vi "Noise_Out_DI.vi"(5 "D2":bool, 6 "D1":bool, 7 "IN":dbl(slide) scale=0.0..9000.0) -> (0 "cluster":cluster{"[0]":dbl, "[1]":dbl}, 1 "DOUT_2":bool, 2 "DOUT_1":bool, 3 "OUT":u32)   [LabVIEW 2017]
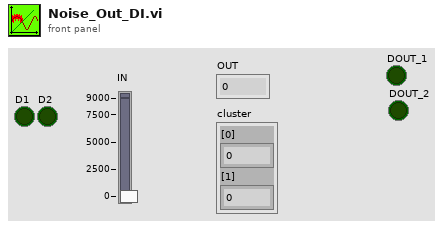
[diagram p1: front panel]
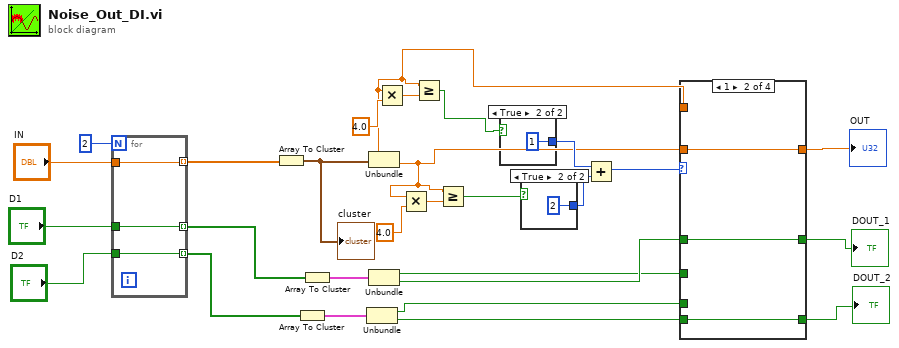
[diagram p0: block diagram]
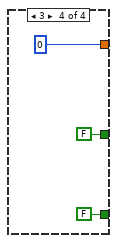
[diagram p4: hidden frame]
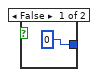
[diagram p5: hidden frame]
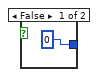
[diagram p6: hidden frame]
diagram:
  n1 = for {
    N: 2 -> [_]
    tunnel: [w31] -> w21 mode=indexing
    tunnel: "IN" -> [w31]
    tunnel: [w30] -> w18 mode=indexing
    tunnel: "D1" -> [w30]
    tunnel: [w29] -> w17 mode=indexing
    tunnel: "D2" -> [w29]
  }
  n2 = Array To Cluster(array=w21) -> (cluster=w28:cluster{"[0]":dbl, "[1]":dbl})
  "cluster" <- w28
  n3 = Array To Cluster(array=w17) -> (cluster=w15:cluster{"[0]":bool, "[1]":bool})
  n4 = Array To Cluster(array=w18) -> (cluster=w16:cluster{"[0]":bool, "[1]":bool})
  n5 = Unbundle(w15) -> ("[0]"=w9:bool, "[1]"=w12:bool)
  n6 = Unbundle(w28) -> ("[0]"=w3:dbl, "[1]"=w4:dbl)
  n7 = Unbundle(w16) -> ("[0]"=w10:bool, "[1]"=w13:bool)
  n8 = Multiply(x=w3, y=4.0) -> (x*y=w6:dbl)
  n9 = Multiply(x=w4, y=4.0) -> (x*y=w8:dbl)
  n10 = Greater Or Equal?(x=w3, y=w6) -> (x >= y?=w1:bool)
  n11 = Greater Or Equal?(x=w4, y=w8) -> (x >= y?=w2:bool)
  n12 = case shown="True" w1 {
    tunnel: [0 1] -> w27
    frame False {
    }
    frame True {
    }
  }
  n13 = case shown="True" w2 {
    tunnel: [0 2] -> w26
    frame False {
    }
    frame True {
    }
  }
  n14 = Add(x=w27, y=w26) -> (x+y=w25:i32)
  n15 = case shown="1" w25 {
    tunnel: [w38 w41 w44 0] -> w24
    tunnel: w3 -> [_ _ w44 _]
    tunnel: w4 -> [w38 w41 _ _]
    tunnel: [w37 w40 w43 FALSE ("[0]")] -> w14
    tunnel: w13 -> [w37 w40 _ _]
    tunnel: w12 -> [w36 w39 _ _]
    tunnel: [w36 w39 w42 FALSE ("[0]")] -> w11
    tunnel: w10 -> [_ _ w43 _]
    tunnel: w9 -> [_ _ w42 _]
    frame 0, Default {
    }
    frame 1 {
    }
    frame 2 {
    }
    frame 3 {
    }
  }
  "OUT" <- w24
  "DOUT_1" <- w14
  "DOUT_2" <- w11
